vi "Make Child TestCase for Method.vi"(8 "error in (no error)":errorcluster, 10 "Test Method":T1) -> (0 "error out":errorcluster, 3 "LUnit Test Case V2 out":refnum<class "LUnit Test Case V2.lvclass">)   [LabVIEW 2020, in "LUnit Test Case V2 Test Double Child.lvclass"]
uses:
  LUnit Test Case V2 Test Double Child.lvclass
  LUnit Test Case/LUnit Test Case V2.lvclass
  LUnit Test Case V2 Test Double/Methods.ctl
  LUnit Test Case V2 Test Double/LUnit Test Case V2 Test Double.lvclass
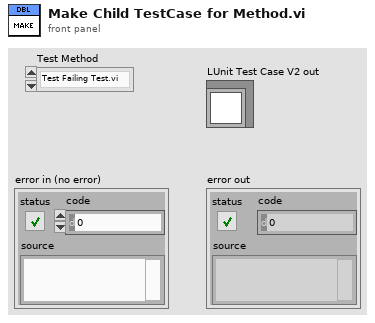
[diagram p1: front panel]
types:
  T1 = typedef "LUnit Test Case V2 Test Double.lvclass/Methods.ctl" = enum16{"Test Failing Test.vi", "Test Passing Test.vi"}
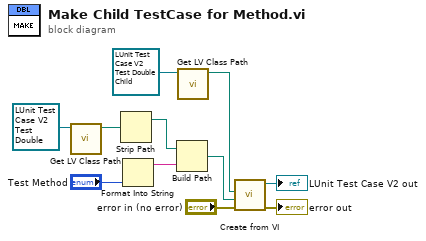
[diagram p0: block diagram]
diagram:
  n1 = call <vilib>:"Get LV Class Path.vi"("object"=refnum<class "LUnit Test Case V2 Test Double.lvclass"> refnum ("LUnit Test Case V2 Test Double.lvclass")) -> ("class path"=w6:path)  [unwired: 9 in, 1 out]
  n2 = Strip Path(path=w6) -> (stripped path=w5:path)  [unwired: 1 out]
  n3 = Format Into String("Test Method") -> (resulting string=w4:string)  [unwired: 3 in, 1 out]
  n4 = Build Path(base path=w5, name or relative path=w4) -> (appended path=w11:path)
  n5 = call <vilib>:"Get LV Class Path.vi"("object"=refnum<class "LUnit Test Case V2 Test Double Child.lvclass"> refnum ("LUnit Test Case V2 Test Double Child.lvclass")) -> ("class path"=w1:path)  [unwired: 9 in, 1 out]
  n6 = call "Create from VI.vi"("error in (no error)"="error in (no error)", "Test Method VI Path"=w11, "Test Case LVCLass Path"=w1) -> ("error out"=→"error out":errorcluster, "LUnit Test Case V2 out"=→"LUnit Test Case V2 out":refnum<class "LUnit Test Case V2.lvclass">)  [unwired: 7 in]
